vi "Service.vi"(8 "error in":errorcluster, 9 "Data":u8[](array[numeric]) format="%.0x", 10 "COB ID":u32 format="%.0x", 11 "CAN Task in":refnum<class "CAN Task.lvclass">) -> (0 "error out":errorcluster, 2 "Processed?":bool, 3 "CAN Task out":refnum<class "CAN Task.lvclass">)   [LabVIEW 2024, in "canopen.lvlib" / "CAN Task.lvlib" / "CAN Task.lvclass"]
uses:
  CAN Task.lvclass
  CAN Task.lvclass/CAN Task.ctl
  CANopen.lvclass
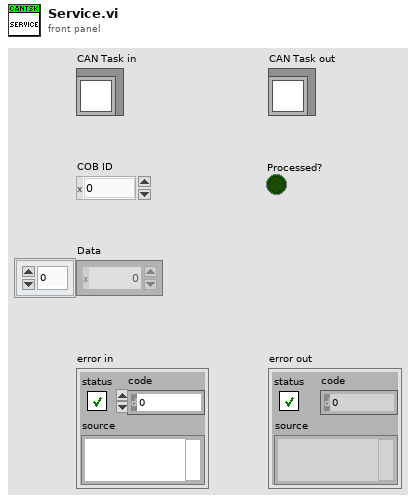
[diagram p1: front panel]
types:
  T1 = cluster{"CobID":u32, "Data offset":u8, "Data size":u8, "Destination":refnum<vi>}[]
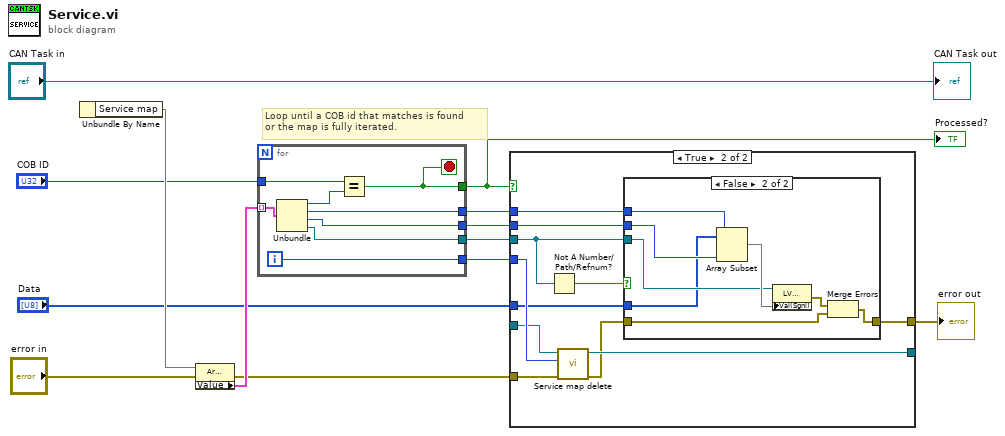
[diagram p0: block diagram]
diagram:
  # "Loop until a COB id that matches is found\nor the map is fully iterated."
  n1 = Unbundle By Name() -> ("Service map"=w9)  [unwired: 1 in]
  n2 = property class="Arr (strict)"(reference=w9, error in="error in") -> (error out=w11:errorcluster, "Value"=w12:T1)  [unwired: 1 out]
  n3 = for {
    tunnel: w12 -> [w22] mode=indexing
    tunnel: [w20] -> w3
    tunnel: [w19] -> w13
    tunnel: [w18] -> w8
    tunnel: [w17] -> w7
    tunnel: [w16] -> w6
    tunnel: "COB ID" -> [w15]
    i -> [w19]
    stop <- w20 stop-if-true
    n4 = Unbundle(w22) -> ("CobID"=w21:u32, "Data offset"=w16:u8, "Data size"=w18:u8, "Destination"=w17:refnum<vi>)
    n5 = Equal?(x=w15, y=w21) -> (x = y?=w20:bool)
  }
  "Processed?" <- w3
  n6 = case shown="True" w3 {
    tunnel: w13 -> [_ w34]
    tunnel: w11 -> [w24 w35]
    tunnel: [w24 w27] -> w4
    tunnel: [w23 w33] -> _
    tunnel: [w23 w32] -> w10
    tunnel: w8 -> [_ w30]
    tunnel: w7 -> [_ w28]
    tunnel: w6 -> [_ w31]
    tunnel: "Data" -> [_ w25]
    frame False {
    }
    frame True {
      n7 = Not A Number/Path/Refnum?(number/path/refnum=w28) -> (NaN/Path/Refnum?=w29:bool)
      n8 = call "Service map delete.vi"("error in (no error)"=w35, "Index"=w34, "CANopen in"=w32) -> ("error out"=w26:errorcluster, "CANopen out"=w33:refnum<class "CANopen.lvclass">)  [unwired: 3 out]
      n9 = case shown="False" w29 {
        tunnel: [w36 w41] -> w27
        tunnel: w31 -> [_ w44]
        tunnel: w30 -> [_ w43]
        tunnel: w28 -> [_ w38]
        tunnel: w26 -> [w36 w40]
        tunnel: w25 -> [_ w37]
        frame True {
        }
        frame False {
          n10 = Array Subset(array=w37, index=w44, length=w43) -> (w39:u8[])
          n11 = property class="LVVar"(reference=w38, "Val(Sgnl)"=w39) -> (error out=w42:errorcluster)  [unwired: 1 in, 1 out]
          n12 = Merge Errors(w42, w40) -> (w41:errorcluster)
        }
      }
    }
  }
  "error out" <- w4
  "CAN Task out" <- "CAN Task in"
